vi "solar_excel Open.vi"(8 "error in (no error)":errorcluster, 9 "Visible? (F)":bool, 10 "Open New Instance? (F)":bool) -> (0 "error out":errorcluster, 3 "Excel App":T1)   [LabVIEW 2018]
doc: "This opens an Excel Application reference."
uses:
  solar_excel_ctl App.ctl
  solar_excel_ctl TSV.ctl
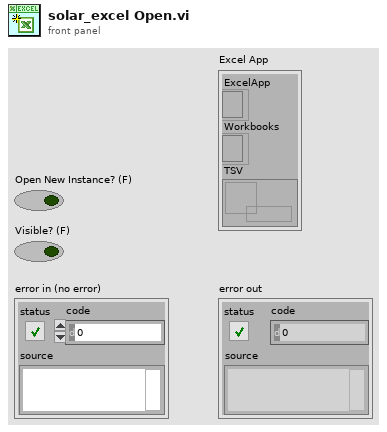
[diagram p1: front panel]
types:
  T1 = typedef "solar_excel_ctl App.ctl" = cluster{"ExcelApp":refnum<k7>, "Workbooks":refnum<k7>, "TSV":refnum<queue>}
  T2 = typedef "solar_excel_ctl TSV.ctl" = cluster{"Path":path, "Dirty":bool, "ActiveSheet":u8, "Worksheets":string[], "Worksheet Cells":cluster{"Cells":string[][]}[]}
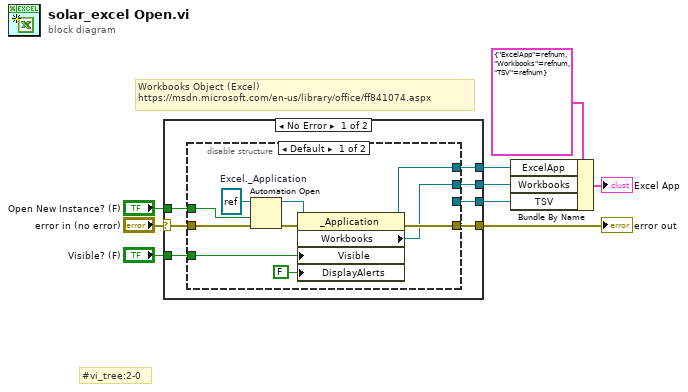
[diagram p0: block diagram]
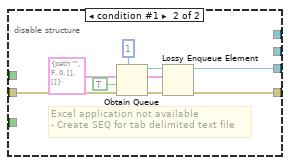
[diagram p2: hidden frame]
diagram:
  # "#vi_tree:2-0"
  # "Workbooks Object (Excel)\nhttps://msdn.microsoft.com/en-us/library/office/ff841074.aspx"
  n1 = case shown="No Error" "error in (no error)" {
    selector: "error in (no error)" -> [w16 w35]
    tunnel: [w15 w35] -> w9
    tunnel: "Visible? (F)" -> [w14 _]
    tunnel: [w13 _] -> w5
    tunnel: [w12 _] -> w4
    tunnel: "Open New Instance? (F)" -> [w11 _]
    tunnel: [w10 _] -> w1
    frame No Error {
      n2 = disable-structure shown="Default" {
        disable-tunnel: w16 -> [w26 w34]
        disable-tunnel: [w23 w28] -> w15
        disable-tunnel: w14 -> [w21 _]
        disable-tunnel: [w19 _] -> w13
        disable-tunnel: [w18 _] -> w12
        disable-tunnel: w11 -> [w17 _]
        disable-tunnel: [_ w27] -> w10
        frame condition #0 (active) {
          w24 = refnum<k7> refnum  # Excel._Application
          n3 = Automation Open(error in (no error)=w26, Automation Refnum=w24, 9:w17) -> (Automation Refnum=w22:refnum<k7>, error out=w25:errorcluster)  [unwired: 1 in]
          n4 = property class="_Application"(reference=w22, error in=w25, "Visible"=w21, "DisplayAlerts"=FALSE) -> (reference out=w19:refnum<k7>, error out=w23:errorcluster, "Workbooks"=w18:refnum<k7>)
        }
        frame condition #1 {
          w29 = T2 {"Path"=path "", "Dirty"=FALSE, "ActiveSheet"=0, "Worksheets"=[], "Worksheet Cells"=[]} ("TSV")
          # "Excel application not available\n- Create SEQ for tab delimited text file"
          n5 = Obtain Queue(max queue size (-1, unlimited)=1, element data type=w29, create if not found? (T)=TRUE, error in (no error)=w34) -> (queue out=w31:refnum<queue>, error out=w30:errorcluster)  [unwired: 1 in, 1 out]
          n6 = Lossy Enqueue Element(queue=w31, element=w29, error in (no error)=w30) -> (queue out=w27:refnum<queue>, error out=w28:errorcluster)  [unwired: 2 out]
        }
      }
    }
    frame Error {
    }
  }
  "error out" <- w9
  n7 = Bundle By Name(cluster=T1 {"ExcelApp"=refnum, "Workbooks"=refnum, "TSV"=refnum} ("ExcelApp 2"), "ExcelApp"=w5, "Workbooks"=w4, "TSV"=w1) -> (→"Excel App":T1)
